vi "DBLtoMenuItem.vi"(8 "error in (no error)":errorcluster, 10 "Double In":dbl, 11 "MenuCol in":refnum<class "MenuCol.lvclass">) -> (0 "error out":errorcluster, 2 "Menu Item":string, 3 "MenuCol out":refnum<class "MenuCol.lvclass">)   [LabVIEW 2013, in "MenuCol.lvclass"]
doc: "Converts an input double to the string corresponding to the menu item of the nearest integer index. Throws an error if the input value is <0 or larger than the greatest index."
uses:
  MenuCol.lvclass
  <vilib>/Utility/error.llb/DialogType.ctl
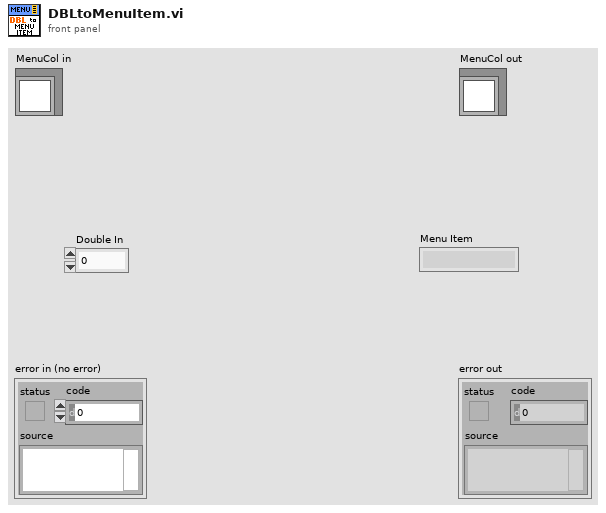
[diagram p1: front panel]
types:
  T1 = typedef "DialogType.ctl" = u16
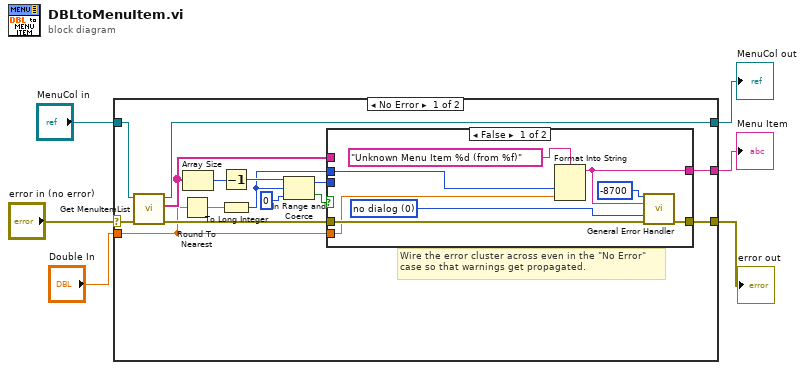
[diagram p0: block diagram]
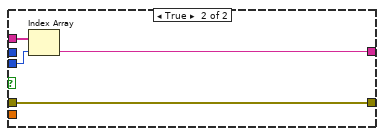
[diagram p2: hidden frame]
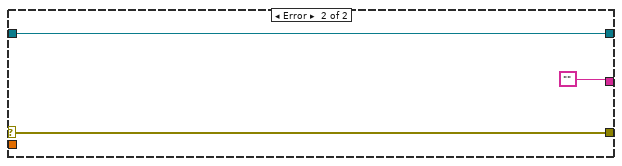
[diagram p3: hidden frame]
diagram:
  n1 = case shown="No Error" "error in (no error)" {
    selector: "error in (no error)" -> [w11 w36]
    tunnel: [w10 w36] -> w5
    tunnel: [w20 w35] -> w3
    tunnel: "MenuCol in" -> [w21 w35]
    tunnel: [w9 ""] -> w2
    tunnel: "Double In" -> [w8 _]
    frame No Error {
      # "Wire the error cluster across even in the \"No Error\"\ncase so that warnings get propagated."
      n2 = call-dynamic "Get MenuItemList.vi"("error in (no error)"=w11, "MenuCol in"=w21) -> ("error out"=w12:errorcluster, "MenuItemList"=w13:string[], "MenuCol out"=w20:refnum<class "MenuCol.lvclass">)  [unwired: 7 in]
      n3 = Round To Nearest(number=w8) -> (nearest integer value=w16:dbl)
      n4 = Array Size(array=w13) -> (size(s)=w19:i32)
      n5 = Decrement(x=w19) -> (x-1=w18:i32)
      n6 = To Long Integer(number=w16) -> (32bit integer=w7:i32)
      n7 = In Range and Coerce(upper limit=w18, x=w7, lower limit=0) -> (coerced(x)=w14:i32, In Range?=w15:bool)
      n8 = case shown="False" w15 {
        tunnel: w14 -> [_ w33]
        tunnel: w13 -> [_ w32]
        tunnel: w12 -> [w29 w31]
        tunnel: [w28 w31] -> w10
        tunnel: [w24 w30] -> w9
        tunnel: w8 -> [w23 _]
        tunnel: w7 -> [w22 _]
        frame False {
          w27 = T1 0 items=["no dialog", "OK message", "continue or stop message", "OK message + warnings", "continue/stop + warnings"] ("type of dialog (OK msg:1)")
          n9 = Format Into String(format string="Unknown Menu Item %d (from %f)" ("String"), w22, w23) -> (resulting string=w24:string)  [unwired: 2 in, 1 out]
          n10 = call <vilib>:"General Error Handler.vi"("[error code] (0)"=-8700, "[error source] (\" \")"=w24, "type of dialog (OK msg:1)"=w27, "error in (no error)"=w29) -> ("error out"=w28:errorcluster)  [unwired: 7 in, 4 out]
        }
        frame True {
          n11 = Index Array(array=w32, index=w33) -> (element=w30:string)
        }
      }
    }
    frame Error {
    }
  }
  "error out" <- w5
  "MenuCol out" <- w3
  "Menu Item" <- w2
